vi "Init Events.vi"(8 "error in (no error)":errorcluster, 11 "Dynamic Combobox in":refnum<class "Dynamic Combobox.lvclass">) -> (0 "error out":errorcluster, 3 "Dynamic Combobox out":refnum<class "Dynamic Combobox.lvclass">, 5 "External Events":T1)   [LabVIEW 2020, in "Dynamic Combobox.lvlib" / "Dynamic Combobox.lvclass"]
uses:
  Dynamic Combobox.lvclass
  Dynamic Combobox Events.ctl
  Dynamic Combobox.lvclass/Dynamic Combobox.ctl
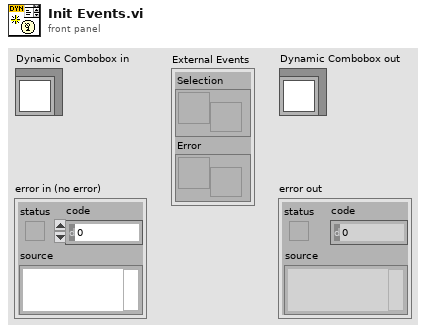
[diagram p1: front panel]
types:
  T1 = typedef "Dynamic Combobox.lvlib/Dynamic Combobox.lvclass/Dynamic Combobox Events.ctl" = cluster{"Selection":refnum<user-event>, "Error":refnum<user-event>}
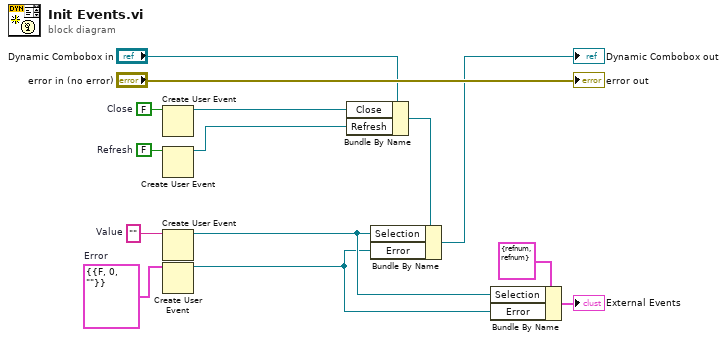
[diagram p0: block diagram]
diagram:
  w2 = cluster{"Error":errorcluster} {"Error"={"status"=FALSE, "code"=0, "source"=""}}  # Error
  w8 = ""  # Value
  w11 = FALSE  # Refresh
  w13 = FALSE  # Close
  n1 = Create User Event(user event datatype=w13) -> (user event=w12:refnum<user-event>)  [unwired: 1 in, 1 out]
  n2 = Create User Event(user event datatype=w11) -> (user event=w9:refnum<user-event>)  [unwired: 1 in, 1 out]
  n3 = Create User Event(user event datatype=w8) -> (user event=w4:refnum<user-event>)  [unwired: 1 in, 1 out]
  n4 = Create User Event(user event datatype=w2) -> (user event=w1:refnum<user-event>)  [unwired: 1 in, 1 out]
  n5 = Bundle By Name(cluster="Dynamic Combobox in", "Close"=w12, "Refresh"=w9) -> (w7:refnum<class "Dynamic Combobox.lvclass">)
  n6 = Bundle By Name(cluster=w7, "Selection"=w4, "Error"=w1) -> (→"Dynamic Combobox out":refnum<class "Dynamic Combobox.lvclass">)
  n7 = Bundle By Name(cluster=T1 {"Selection"=refnum, "Error"=refnum} ("Dynamic Combobox Events"), "Selection"=w4, "Error"=w1) -> (→"External Events":T1)
  "error out" <- "error in (no error)"
